vi "Set Detection.vi"(8 "error in (no error)":errorcluster, 9 "Optical Path":T1=1 items=["Eyepieces"=1, "Right"=2, "Bottom"=3, "Left"=4], 10 "Filter Position":T2=1 items=["1"=1, "2"=2, "3"=3, "4"=4, "5"=5, "6"=6], 11 "Microscope In":refnum<class "Nikon Stand.lvclass">) -> (0 "error out":errorcluster, 3 "Microscope Out":refnum<class "Nikon Stand.lvclass">)   [LabVIEW 2023, in "Nikon Stand.lvlib" / "Nikon Stand.lvclass"]
uses:
  Nikon Stand.lvclass
  Microscope/ti2lv/ti2_filterPos.ctl
  Microscope/ti2lv/ti2_lightPath.ctl
  Microscope/ti2lv/ti2lv.lvlib
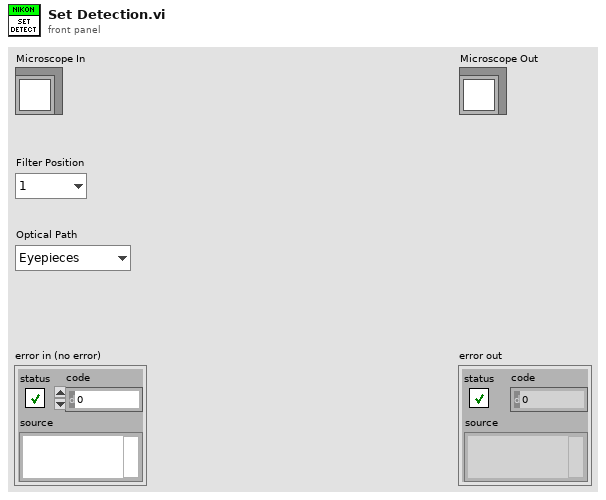
[diagram p1: front panel]
types:
  T1 = typedef "ti2lv.lvlib/ti2_lightPath.ctl" = i32
  T2 = typedef "ti2lv.lvlib/ti2_filterPos.ctl" = u16
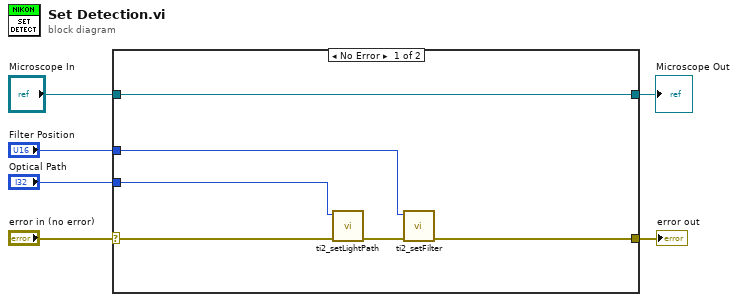
[diagram p0: block diagram]
diagram:
  n1 = case shown="No Error" "error in (no error)" {
    selector: "error in (no error)" -> [w12 w14]
    tunnel: [w11 w14] -> w5
    tunnel: [w8 w13] -> w1
    tunnel: "Microscope In" -> [w8 w13]
    tunnel: "Optical Path" -> [w10 _]
    tunnel: "Filter Position" -> [w9 _]
    frame No Error {
      n2 = call "ti2_setLightPath.vi"("error in (no error)"=w12, "Light Path"=w10) -> ("error out"=w7:errorcluster)  [unwired: 9 in]
      n3 = call "ti2_setFilter.vi"("error in (no error)"=w7, "Filter Position"=w9) -> ("error out"=w11:errorcluster)  [unwired: 9 in]
    }
    frame Error {
    }
  }
  "error out" <- w5
  "Microscope Out" <- w1
